vi "Verify Chan Volt Cal Test from ALL CHANNELS DATA.vi"(5 "Channel Values":i32[](array[numeric]), 6 "calbuffer":u8[](array[numeric]), 8 "error in (no error)":errorcluster, 9 "Scale":T1, 11 "Channel Number (1-4)":i32=1 min=1 max=4) -> (0 "error out":errorcluster, 3 "Channel Voltage Result":dbl)   [LabVIEW 2015]
uses:
  DLL/Scales.ctl
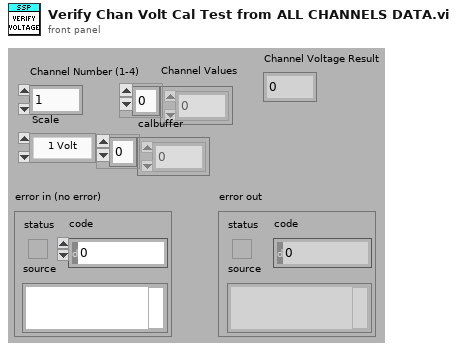
[diagram p1: front panel]
types:
  T1 = typedef "Scales.ctl" = enum16{"1 Volt", "2 Volt", "5 Volt", "10 Volt", "20 Volt", "50 Volt", "100 Volt", "200 Volt", "400 Volt"}
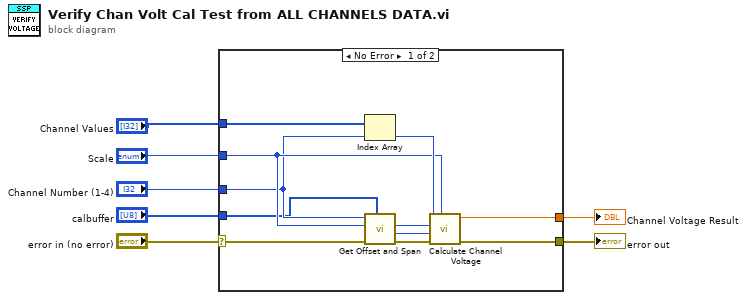
[diagram p0: block diagram]
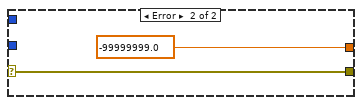
[diagram p2: hidden frame]
diagram:
  n1 = case shown="No Error" "error in (no error)" {
    selector: "error in (no error)" -> [w11 w20]
    tunnel: [w18 w20] -> w7
    tunnel: "Channel Values" -> [w17 _]
    tunnel: "Channel Number (1-4)" -> [w14 _]
    tunnel: "Scale" -> [w15 _]
    tunnel: [w9 -99999999.0 ("Channel Voltage Result")] -> w2
    tunnel: "calbuffer" -> [w8 _]
    frame No Error {
      n2 = Index Array(array=w17, index=w14) -> (element=w16:i32)
      n3 = call "Get Offset and Span.vi"("calbuffer"=w8, "error in (no error)"=w11, "nScale"=w15, "nWhichChan"=w14) -> ("error out"=w10:errorcluster, "*pnChanSpanOffset"=w12:u16, "*pnChanZeroOffset"=w13:u16)  [unwired: 5 in]
      n4 = call "Calculate Channel Voltage.vi"("Scale"=w15, "error in (no error)"=w10, "ChanSpanOffset"=w12, "ChanZeroOffset"=w13, "ChanValue"=w16) -> ("error out"=w18:errorcluster, "Channel Voltage Result"=w9:dbl)  [unwired: 5 in]
    }
    frame Error {
    }
  }
  "error out" <- w7
  "Channel Voltage Result" <- w2
